vi "Version--constant.vi"() -> (3 "Version Number":string="unreleased")   [LabVIEW 2020, in "hse-db.lvlib" / "DB-Interface.lvclass"]
doc: "____\nHAMPEL SOFTWARE ENGINEERING v1.4.0 (2023-12-19 09:52)"
uses:
  DB-Interface.lvclass
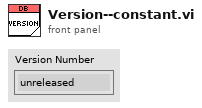
[diagram p1: front panel]
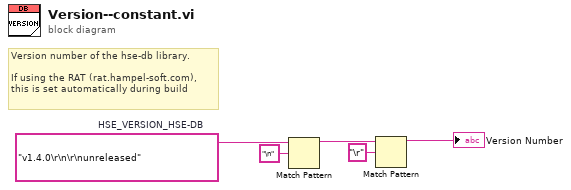
[diagram p0: block diagram]
diagram:
  w4 = "v1.4.0\r\n\r\nunreleased"  # HSE_VERSION_HSE-DB
  # "Version number of the hse-db library.\n\nIf using the RAT (rat.hampel-soft.com),\nthis is set automatically during build"
  n1 = Match Pattern(string=w4, regular expression="\n") -> (before substring=w2:string)  [unwired: 1 in, 3 out]
  n2 = Match Pattern(string=w2, regular expression="\r") -> (before substring=→"Version Number":string)  [unwired: 1 in, 3 out]
